vi "Color_Assign.vi"(6 "Add Spaces?":bool, 8 "Front Panel":refnum<vi>, 11 "Code":refnum<vi>) -> (2 "Value":string)   [LabVIEW 2021]
uses:
  <vilib>/Utility/miscctls.llb/LVSelectionTypeDef.ctl
  Color_Globals.vi
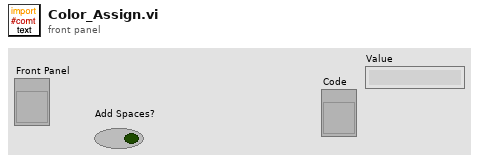
[diagram p1: front panel]
types:
  T1 = typedef "LVSelectionTypeDef.ctl" = cluster{"Selection Start":u32, "Selection End":u32}
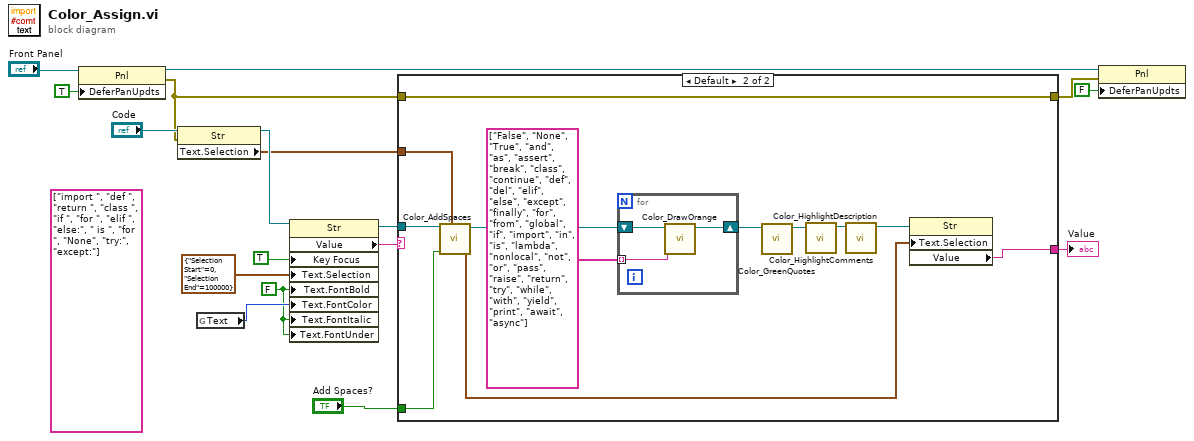
[diagram p0: block diagram]
diagram:
  (unwired) string[] ["import ", "def ", "return ", "class ", "if ", "for ", "elif ", "else:", " is ", "for ", "None", "try:", "except:"]
  w1 = FALSE ("Text.Font:Bold")
  n1 = property class="Pnl"(reference="Front Panel", "DeferPanUpdts"=TRUE ("Defer Panel Updates")) -> (reference out=w9:refnum<vi>, error out=w7:errorcluster)  [unwired: 1 in]
  n2 = property on="Property Node" class="Str"(reference="Code", error in=w7) -> (reference out=w15:refnum<vi>, "Text.Selection"=w14:T1)  [unwired: 1 out]
  n3 = global read "Color_Globals.vi" "Text"() -> (w2:u32)
  n4 = property on="Property Node" class="Str"(reference=w15, "Key Focus"=TRUE, "Text.Selection"=T1 {"Selection Start"=0, "Selection End"=100000}, "Text.FontBold"=w1, "Text.FontColor"=w2, "Text.FontItalic"=w1, "Text.FontUnder"=w1) -> (reference out=w5:refnum<vi>, "Value"=w4:string)  [unwired: 1 in, 1 out]
  n5 = case shown="Default" w4 {
    selector: w4 -> [w19 _]
    tunnel: w5 -> [_ w25]
    tunnel: w14 -> [_ w30]
    tunnel: [w19 w29] -> w12
    tunnel: [w18 w28] -> w8
    tunnel: w7 -> [w18 w28]
    tunnel: "Add Spaces?" -> [_ w26]
    frame "" {
    }
    frame Default {
      n6 = call "Color_AddSpaces.vi"("Text.Selection"=w30, "Add Spaces?"=w26, "String in"=w25) -> ("Cursor"=w27:cluster{u32, u32}, "String out"=w24:refnum<vi>)  [unwired: 7 in]
      n7 = for {
        shift-right: [w33] -> w20
        shift-left: w24 -> [w34]
        tunnel: string[] ["False", "None", "True", "and", "as", "assert", "break", "class", "continue", "def", "del", "elif", "else", "except", "finally", "for", "from", "global", "if", "import", "in", "is", "lambda", "nonlocal", "not", "or", "pass", "raise", "return", "try", "while", "with", "yield", "print", "await", "async"] -> [w32] mode=indexing
        n8 = call "Color_DrawOrange.vi"("Expression"=w32, "String in"=w34) -> ("String out"=w33:refnum<vi>)  [unwired: 9 in]
      }
      n9 = call "Color_GreenQuotes.vi"("String in"=w20) -> ("String out"=w21:refnum<vi>)  [unwired: 10 in]
      n10 = call "Color_HighlightComments.vi"("String in"=w21) -> ("String out"=w22:refnum<vi>)  [unwired: 10 in]
      n11 = call "Color_HighlightDescription.vi"("String in"=w22) -> ("String out"=w23:refnum<vi>)  [unwired: 10 in]
      n12 = property on="Property Node" class="Str"(reference=w23, "Text.Selection"=w27) -> ("Value"=w29:string)  [unwired: 1 in, 2 out]
    }
  }
  "Value" <- w12
  n13 = property class="Pnl"(reference=w9, error in=w8, "DeferPanUpdts"=FALSE ("Defer Panel Updates")) -> ()  [unwired: 2 out]
